vi "test_Create MetaData Channel_array type cast.vi"(8 "error in (no error)":errorcluster, 11 "TestCase in":refnum<class "Instrument Addon Scripting API Channels Unit Tests.lvclass">) -> (0 "error out":errorcluster, 3 "TestCase out":refnum<class "Instrument Addon Scripting API Channels Unit Tests.lvclass">)   [LabVIEW 2019, in "Instrument Addon Scripting API Channels Unit Tests.lvclass"]
uses:
  Instrument Addon Scripting API Channels Unit Tests.lvclass
  Addon/Addon Shared/Types/FG Control.ctl
  APIs/Scripting API/TypeDefs/Array Type Cast Settings.ctl
  APIs/Scripting API/TypeDefs/Array Element.ctl
  Addon/Addon Shared/Types/Type Cast Type.ctl
  Addon/Addon Shared/Types/Endian.ctl
  Instrument Addon Scripting API Channels Unit Tests.lvclass/Instrument Addon Scripting API Channels Unit Tests.ctl
  Addon/Addon Shared/SubVIs/Constants.vi
  <vilib>/NI VeriStand/Custom Device Tools/Custom Device Utility Library/NI VeriStand - Search for Item by Name.vi
  APIs/Scripting API/Channels/Create MetaData Channel - Array - Type Cast.vi
  <vilib>/NI VeriStand/Custom Device Tools/Custom Device Utility Library/NI VeriStand - Search for Item by GUID.vi
  <vilib>/NI VeriStand/Custom Device API/NI VeriStand - Get Item Property.vi
  <vilib>/NI VeriStand/Custom Device API/Get Item Property (U32).vi
  <vilib>/NI VeriStand/Custom Device API/Get Item Property (String Array).vi
  <vilib>/NI VeriStand/Custom Device API/Get Item Property (String).vi
  <vilib>/NI VeriStand/Custom Device API/NI VeriStand - Set Item Property.vi
  <vilib>/NI VeriStand/Custom Device API/Set Item Property (U32).vi
  <vilib>/NI VeriStand/Custom Device API/Set Item Property (String Array).vi
  <vilib>/NI VeriStand/Custom Device API/NI VeriStand - Get Item Children.vi
  Addon/Addon Shared/SubVIs/Set Channel Value Table.vi
  <vilib>/NI VeriStand/Custom Device API/Set Item Property (String).vi
  <vilib>/addons/_JKI Toolkits/VI Tester/TestCase.llb/TestCase.lvclass
  Instrument Addon Scripting API Test Assets/Instrument Addon Scripting API Test Assets.lvclass
  <vilib>/NI VeriStand/Custom Device Tools/Custom Device Utility Library/Custom Device Utility Library.lvlib
  Addon/Addon Shared/Instrument Addon Shared.lvlib
  APIs/Scripting API/Instrument Addon Scripting API.lvlib
  C:/Program Files (x86)/National Instruments/LabVIEW 2019/vi.lib/addons/_JKI Toolkits/VI Tester/TestCase.llb/TestCase.lvclass
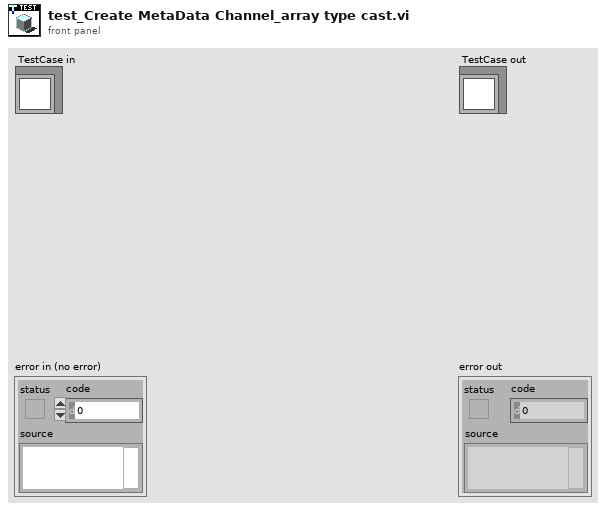
[diagram p1: front panel]
types:
  T1 = typedef "Instrument Addon Shared.lvlib/FG Control.ctl" = enum16{"Get", "Set"}
  T2 = typedef "Instrument Addon Scripting API.lvlib/Array Type Cast Settings.ctl" = cluster{"Elements":T3[], "Delimiter":string, "Type":T4, "Endian":T5}
  T3 = typedef "Instrument Addon Scripting API.lvlib/Array Element.ctl" = cluster{"Name":string, "Default Value":dbl, "Units":string}
  T4 = typedef "Instrument Addon Shared.lvlib/Type Cast Type.ctl" = enum16{"DBL", "SGL", "U64", "U32", "U16", "U8", "I64", "I32", "I16", "I8"}
  T5 = typedef "Instrument Addon Shared.lvlib/Endian.ctl" = enum16{"Native", "Little", "Big"}
  T6 = typedef "Custom Device API.lvlib/Custom Device Item Ref.ctl" = u64
  T7 = typedef "Instrument Addon Shared.lvlib/MetaData Parameters.ctl" = cluster{"Data Type":T8, "Channel Type":T9, "List":string[], "Format String":string, "Type":T4, "Delimiter":string, "Endian":T5}
  T8 = typedef "Instrument Addon Shared.lvlib/Protocol Data Type.ctl" = enum16{"Single Channel", "Array"}
  T9 = typedef "Instrument Addon Shared.lvlib/Metadata Channel Type.ctl" = enum16{"Enumerated List", "Format", "Type Cast"}
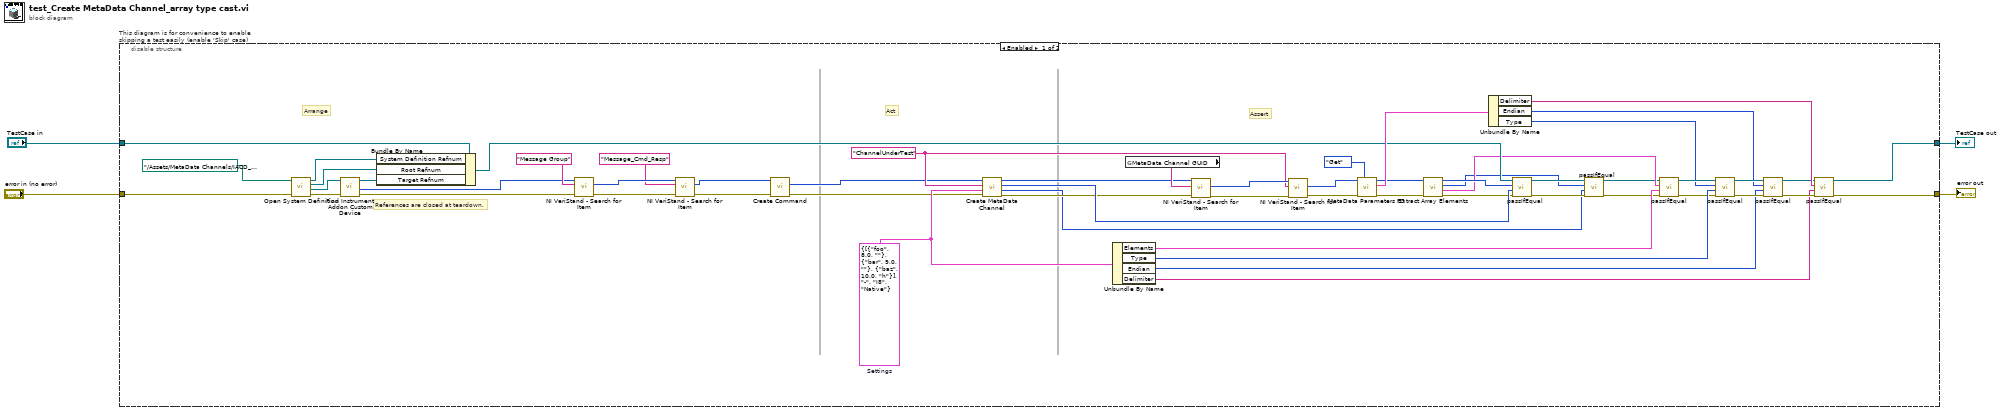
[diagram p0: block diagram]
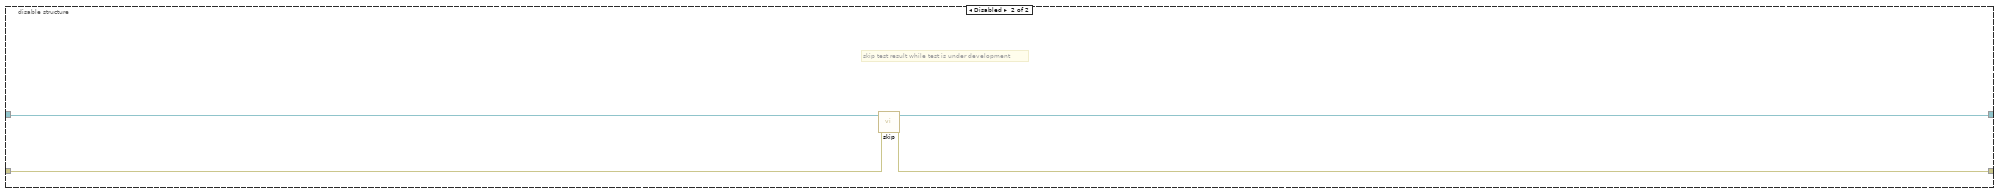
[diagram p2: hidden frame]
diagram:
  n1 = disable-structure "This diagram is for convenience to enable skipping a test easily (enable 'Skip' case)" shown="Enabled" {
    disable-tunnel: "TestCase in" -> [w46 w65]
    disable-tunnel: [w40 w63] -> w1
    disable-tunnel: [w39 w64] -> w3
    disable-tunnel: "error in (no error)" -> [w61 w62]
    frame Enabled {
      w31 = T2 {"Elements"=[{"Name"="foo", "Default Value"=8.0, "Units"=""}, {"Name"="bar", "Default Value"=9.0, "Units"=""}, {"Name"="baz", "Default Value"=10.0, "Units"="h"}], "Delimiter"="-", "Type"=enum."I8", "Endian"=enum."Native"}  # Settings
      w45 = "ChannelUnderTest" ("Name")
      # "References are closed at teardown."
      # "Assert"
      # "Act"
      # "Arrange"
      n2 = call "Open System Definition.vi"("error in (no error)"=w61, "System Definition File"=path "../Assets/MetaData Channels/IACD_channels.nivssdf") -> ("error out"=w59:errorcluster, "Target Refnum"=w60:refnum<k24>, "Root Refnum"=w49:refnum<k24>, "System Definition Refnum"=w48:refnum<k24>)  [unwired: 6 in]
      n3 = call "Find Instrument Addon Custom Device.vi"("error in"=w59, "target in"=w60) -> ("error out"=w17:errorcluster, "NodeID"=w18:u64, "target out"=w50:refnum<k24>)  [unwired: 7 in]
      n4 = Bundle By Name(cluster=w46, "System Definition Refnum"=w48, "Root Refnum"=w49, "Target Refnum"=w50) -> (w47:refnum<class "Instrument Addon Scripting API Channels Unit Tests.lvclass">)
      n5 = call-poly <vilib>:"NI VeriStand - Search for Item.vi"("error in"=w17, "Item Name"="Message Group", "Section Ref in"=w18) -> ("error out"=w19:errorcluster, "Item Ref"=w21:T6)  [unwired: 5 in, 2 out]
      n6 = call-poly <vilib>:"NI VeriStand - Search for Item.vi"("error in"=w19, "Item Name"="Message_Cmd_Resp", "Section Ref in"=w21) -> ("error out"=w8:errorcluster, "Item Ref"=w7:T6)  [unwired: 5 in, 2 out]
      n7 = call "Create Command.vi"("error in"=w8, "message refnum In"=w7) -> ("error out"=w5:errorcluster, "command refnum"=w6:T6)  [unwired: 7 in, 1 out]
      n8 = call-poly "Create MetaData Channel.vi"("error in (no error)"=w5, "settings"=w31, "channel name"=w45, "command refnum in"=w6) -> ("error out"=w42:errorcluster, "channel refnums"=w10:T6[], "array refnum"=w43:T6, "command refnum out"=w44:T6)  [unwired: 4 in]
      n9 = Unbundle By Name(w31) -> ("Elements"=w36:T3[], "Type"=w51:T4, "Endian"=w26:T5, "Delimiter"=w23:string)
      n10 = global read "Constants.vi" "MetaData Channel GUID"() -> (w58:string)
      n11 = call-poly <vilib>:"NI VeriStand - Search for Item.vi"("error in"=w42, "Item GUID"=w58, "Section Ref in"=w44) -> ("error out"=w56:errorcluster, "Item Ref"=w57:T6)  [unwired: 5 in, 2 out]
      n12 = call-poly <vilib>:"NI VeriStand - Search for Item.vi"("error in"=w56, "Item Name"=w45, "Section Ref in"=w57) -> ("error out"=w55:errorcluster, "Item Ref"=w54:T6)  [unwired: 5 in, 2 out]
      n13 = call "MetaData Parameters FG.vi"("Action"=FG_Control."Get", "error in (no error)"=w55, "Item Ref in"=w54) -> ("error out"=w35:errorcluster, "MetaData Parameters"=w52:T7, "Item Ref out"=w34:T6)  [unwired: 6 in]
      n14 = call "Extract Array Elements.vi"("error in (no error)"=w35, "array reference in"=w34) -> ("error out"=w33:errorcluster, "elements"=w16:T3[], "channel refnums"=w11:T6[], "array reference out"=w32:T6)  [unwired: 6 in]
      n15 = Unbundle By Name(w52) -> ("Delimiter"=w41:string, "Endian"=w24:T5, "Type"=w25:T4)
      n16 = call-dynamic "passIfEqual.vi"("error in (no error)"=w33, "y"=w43, "x"=w32, "TestCase in"=w47) -> ("error out"=w14:errorcluster, "TestCase out"=w15:refnum<class "Instrument Addon Scripting API Channels Unit Tests.lvclass">)  [unwired: 6 in]
      n17 = call-dynamic "passIfEqual.vi"("error in (no error)"=w14, "y"=w10, "x"=w11, "TestCase in"=w15) -> ("error out"=w12:errorcluster, "TestCase out"=w13:refnum<class "Instrument Addon Scripting API Channels Unit Tests.lvclass">)  [unwired: 6 in]
      n18 = call-dynamic "passIfEqual.vi"("error in (no error)"=w12, "y"=w36, "x"=w16, "TestCase in"=w13) -> ("error out"=w37:errorcluster, "TestCase out"=w38:refnum<class "Instrument Addon Scripting API Channels Unit Tests.lvclass">)  [unwired: 6 in]
      n19 = call-dynamic "passIfEqual.vi"("error in (no error)"=w37, "y"=w51, "x"=w25, "TestCase in"=w38) -> ("error out"=w29:errorcluster, "TestCase out"=w30:refnum<class "Instrument Addon Scripting API Channels Unit Tests.lvclass">)  [unwired: 6 in]
      n20 = call-dynamic "passIfEqual.vi"("error in (no error)"=w29, "y"=w26, "x"=w24, "TestCase in"=w30) -> ("error out"=w27:errorcluster, "TestCase out"=w28:refnum<class "Instrument Addon Scripting API Channels Unit Tests.lvclass">)  [unwired: 6 in]
      n21 = call-dynamic "passIfEqual.vi"("error in (no error)"=w27, "y"=w23, "x"=w41, "TestCase in"=w28) -> ("error out"=w39:errorcluster, "TestCase out"=w40:refnum<class "Instrument Addon Scripting API Channels Unit Tests.lvclass">)  [unwired: 6 in]
    }
    frame Disabled {
      # "skip test result while test is under development"
      n22 = call <vilib>:"skip.vi"("error in (no error)"=w62, "TestCase in"=w65) -> ("error out"=w64:errorcluster, "TestCase out"=w63:refnum<class "Instrument Addon Scripting API Channels Unit Tests.lvclass">)  [unwired: 8 in]
    }
  }
  "error out" <- w3
  "TestCase out" <- w1
